vi "mqttTCPIPserver.vi"(0 "mqtt.lvclass":refnum<class "mqtt.lvclass">, 11 "error in (no error)":errorcluster) -> (4 "mqtt.lvclass 2":refnum<class "mqtt.lvclass">, 15 "error out":errorcluster)   [LabVIEW 2018, in "labview-mqtt.lvlib" / "mqtt.lvclass"]
uses:
  mqtt.lvclass
  mqtt.lvclass/mqtt.ctl
  mqttTypedef/mqttRXdataCluster.ctl
  mqttTypedef/mqttFixedHeaderResponse.ctl
  mqttTypedef/mqttQOSlevel.ctl
  mqttTypedef/mqttMessageType.ctl
  mqttTypedef/mqttRXsubscriptionEventData.ctl
  labview-mqtt.lvlib
  mqttCmd/mqttCmdPublish/mqttCmdPublish.lvclass
  mqttCmd/mqttCmdPing/mqttCmdPing.lvclass
panel:
  out "rxCount":i32
  out "rxTelegram":u8[](array[numeric]) format="%02x"
  out "txError":errorcluster
  out "txTelegram":u8[](array[numeric]) format="%02x"
  out "payloadError":errorcluster
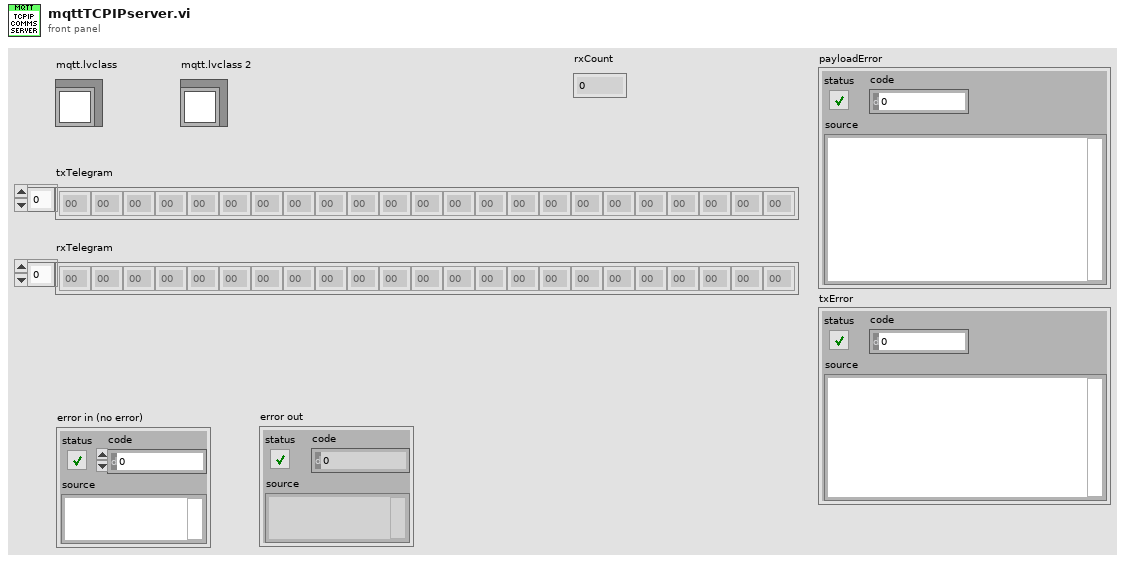
[diagram p1: front panel]
types:
  T1 = typedef "labview-mqtt.lvlib/mqttRXdataCluster.ctl" = cluster{"fixedHdr":T2, "payload":u8[]}
  T2 = typedef "labview-mqtt.lvlib/mqttFixedHeaderResponse.ctl" = cluster{"retain":bool, "qos":T3, "duplicate":bool, "response":T4}
  T3 = typedef "labview-mqtt.lvlib/mqttQOSlevel.ctl" = enum8{"At most once", "At least once", "Exactly once", "Reserved"}
  T4 = typedef "labview-mqtt.lvlib/mqttMessageType.ctl" = enum32{"Reserved", "CONNECT", "CONNACK", "PUBLISH", "PUBACK", "PUBREC", "PUBREL", "PUBCOMP", "SUBSCRIBE", "SUBACK", "UNSUBSCRIBE", "UNSUBACK", "PINGREQ", "PINGRESP", "DISCONNECT", "Reserved2"}
  T5 = typedef "labview-mqtt.lvlib/mqttRXsubscriptionEventData.ctl" = cluster{"topic":string, "value":string, "messageID":u16}
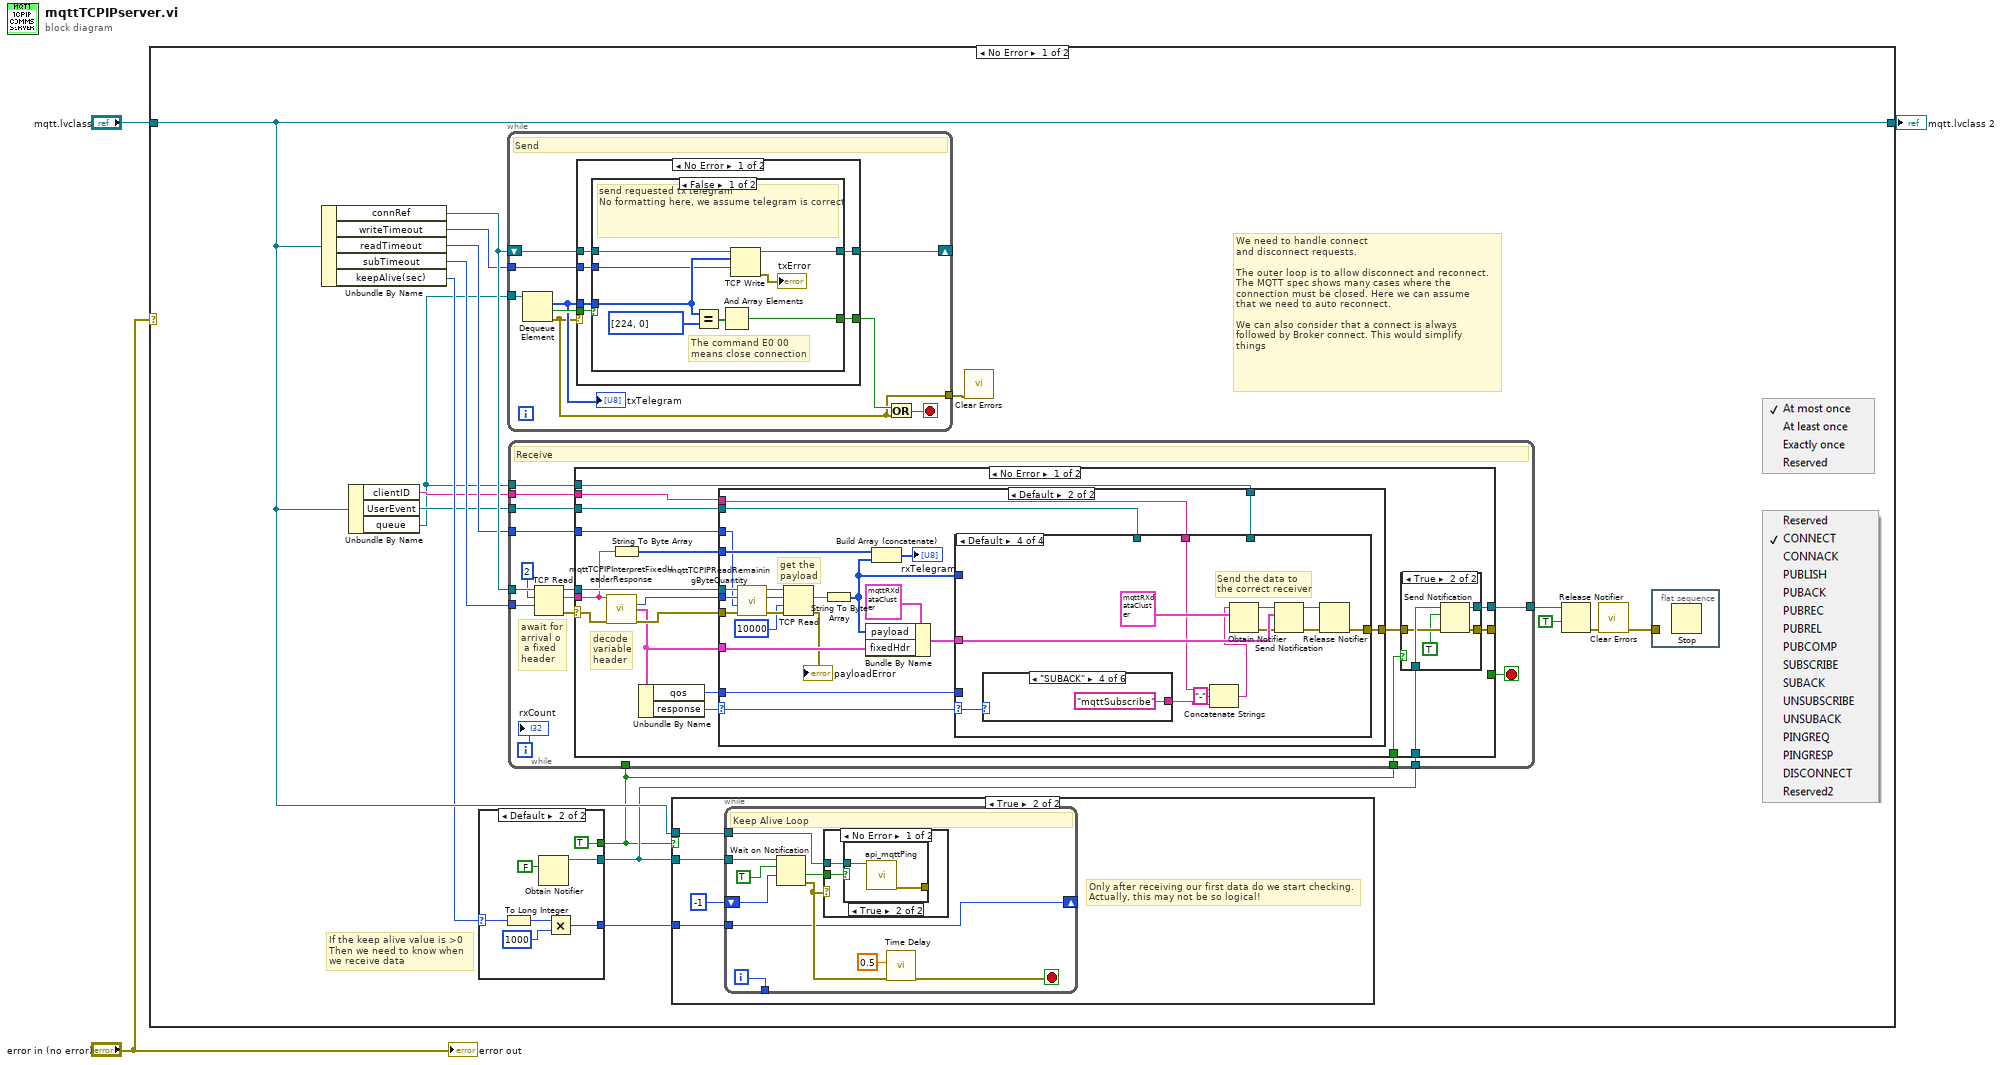
[diagram p0: block diagram]
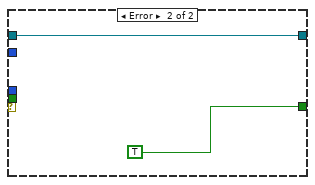
[diagram p7: hidden frame]
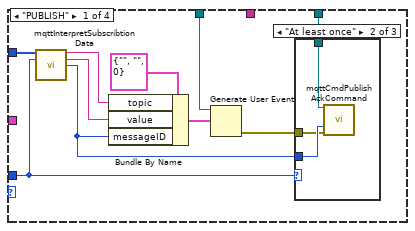
[diagram p10: hidden frame]
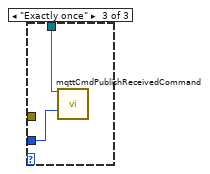
[diagram p12: hidden frame]
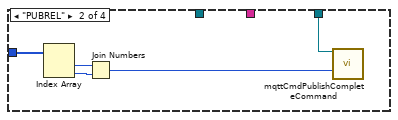
[diagram p13: hidden frame]
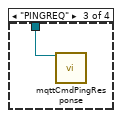
[diagram p14: hidden frame]
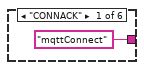
[diagram p15: hidden frame]
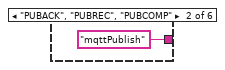
[diagram p16: hidden frame]
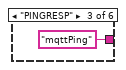
[diagram p17: hidden frame]
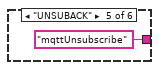
[diagram p18: hidden frame]
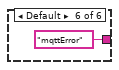
[diagram p19: hidden frame]
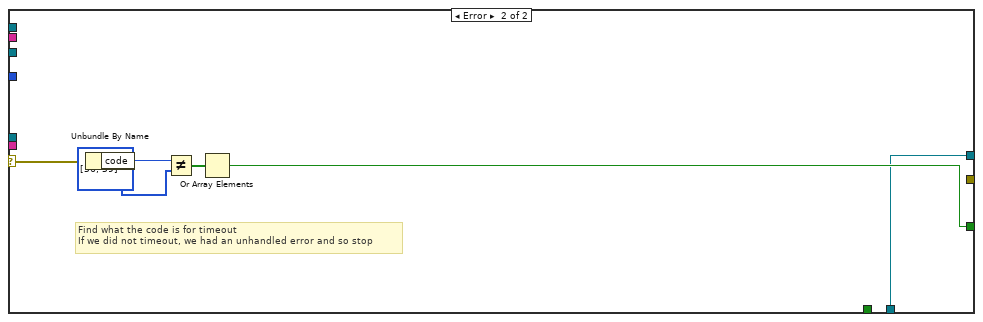
[diagram p20: hidden frame]
diagram:
  n1 = case shown="No Error" "error in (no error)" {
    tunnel: "mqtt.lvclass" -> [w20 w177]
    tunnel: [w20 w177] -> w2
    frame No Error {
      # "If the keep alive value is >0\nThen we need to know when\nwe receive data"
      # "We need to handle connect\nand disconnect requests.\n\nThe outer loop is to allow disconnect and reconnect.\nThe MQTT spec shows many cases where the\nconnection must be closed. Here we can assume\nthat we need to auto reconnect.\n\nWe can also consider that a connect is always\nfollowed by Broker connect. This would simplify\nthings"
      n2 = Unbundle By Name(w20) -> ("connRef"=w19:refnum<k5>, "writeTimeout"=w17:i32, "readTimeout"=w16:i32, "subTimeout"=w15:i32, "keepAlive(sec)"=w9:u16)
      n3 = Unbundle By Name(w20) -> ("clientID"=w6:string, "UserEvent"=w7:refnum<user-event>, "queue"=w5:refnum<queue>)
      n4 = case shown="Default" w9 {
        selector: w9 -> [_ w40]
        tunnel: [_ w45] -> w14
        tunnel: [_ w41] -> w10
        tunnel: [_ TRUE] -> w8
        frame ..0 {
        }
        frame Default {
          n5 = To Long Integer(number=w40) -> (32bit integer=w43:i32)
          n6 = Obtain Notifier(notification data type=FALSE) -> (notifier out=w45:refnum<notifier>)  [unwired: 3 in, 2 out]
          n7 = Multiply(x=w43, y=1000) -> (x*y=w41:i32)
        }
      }
      n8 = while {
        tunnel: w5 -> [w54]
        shift-right: [w51] -> _
        shift-left: w19 -> [w52]
        tunnel: [w47] -> w18
        tunnel: w17 -> [w46]
        stop <- w50 stop-if-true
        # "Send"
        n9 = Dequeue Element(queue=w54) -> (element=w48:u8[], timed out?=w53:bool, error out=w47:errorcluster)  [unwired: 2 in, 1 out]
        "txTelegram" <- w48
        n10 = case shown="No Error" w47 {
          tunnel: w53 -> [w60 _]
          tunnel: w48 -> [w59 _]
          tunnel: w52 -> [w58 w71]
          tunnel: [w57 w71] -> w51
          tunnel: [w56 TRUE] -> w49
          tunnel: w46 -> [w55 _]
          frame No Error {
            n11 = case shown="False" w60 {
              tunnel: w59 -> [w66 _]
              tunnel: w58 -> [w68 w69]
              tunnel: [w67 w69] -> w57
              tunnel: [w63 _] -> w56
              tunnel: w55 -> [w61 _]
              frame False {
                # "The command E0 00\nmeans close connection"
                # "send requested tx telegram\nNo formatting here, we assume telegram is correct"
                n12 = Equal?(x=w66, y=u8[] [224, 0] ("txTelegram 2")) -> (x = y?=w64:bool[])
                n13 = And Array Elements(Boolean array=w64) -> (logical AND=w63:bool)
                n14 = TCP Write(connection ID=w68, data in=w66, 9:w61) -> (connection ID out=w67:refnum<k5>, error out=→"txError":errorcluster)  [unwired: 1 in, 1 out]
              }
              frame True {
                # "Queue Timed Out - do nothing.\nWe can later use this for the Keep Alive ping"
              }
            }
          }
          frame Error {
          }
        }
        n15 = Or(x=w49, y=w47) -> (x .or. y?=w50:bool)
      }
      n16 = while {
        tunnel: w19 -> [w86]
        tunnel: w16 -> [w79]
        tunnel: w15 -> [w78]
        tunnel: w14 -> [w77]
        tunnel: [w76] -> w13
        tunnel: w8 -> [w75]
        tunnel: w8 -> [_]
        tunnel: w7 -> [w74]
        tunnel: w5 -> [w73]
        tunnel: w6 -> [w72]
        i -> [w80]
        stop <- w81 stop-if-true
        # "await for\narrival o\n a fixed\nheader"
        # "Receive"
        n17 = TCP Read(connection ID=w86, bytes to read=2, 9:w78) -> (connection ID out=w85:refnum<k5>, data out=w82:string, error out=w84:errorcluster)  [unwired: 2 in]
        n18 = case shown="No Error" w84 {
          selector: w84 -> [w102 w176]
          tunnel: w85 -> [w103 _]
          tunnel: w82 -> [w98 _]
          tunnel: [_ w172] -> w81
          tunnel: w79 -> [w95 _]
          tunnel: w77 -> [w94 w171]
          tunnel: [w92 w171] -> w76
          tunnel: [w91 _] -> _
          tunnel: w75 -> [w90 _]
          tunnel: w74 -> [w89 _]
          tunnel: w73 -> [w88 _]
          tunnel: w72 -> [w87 _]
          frame No Error {
            # "decode\nvariable\nheader"
            n19 = call "mqttTCPIPInterpretFixedHeaderResponse.vi"("data in"=w98, "error in (no error)"=w102) -> ("remainingLengthByte1"=w104:u8, "output cluster"=w100:T2, "error out"=w101:errorcluster)  [unwired: 11 in]
            n20 = String To Byte Array(string=w98) -> (unsigned byte array=w97:u8[])
            n21 = Unbundle By Name(w100) -> ("qos"=w96:T3, "response"=w99:T4)
            n22 = case shown="Default" w99 {
              selector: w99 -> [_ w121]
              tunnel: w104 -> [_ w131]
              tunnel: w103 -> [_ w130]
              tunnel: w101 -> [_ w123]
              tunnel: w100 -> [_ w122]
              tunnel: w97 -> [_ w118]
              tunnel: w96 -> [_ w117]
              tunnel: w95 -> [_ w114]
              tunnel: [_ w113] -> w93
              tunnel: w89 -> [_ w112]
              tunnel: w88 -> [_ w111]
              tunnel: w87 -> [_ w110]
              frame "CONNECT", "SUBSCRIBE" {
                # "The client should not receive these commands.\nI had some problems with these commands being received\nand it appears this was a broker issue. However, to ignore\nmessages that we should not receive is no bad thing."
              }
              frame Default {
                # "get the\npayload"
                n23 = call "mqttTCPIPReadRemainingByteQuantity.vi"("error in (no error)"=w123, "readTimeout ms (2000)"=w114, "remainingLengthByte1"=w131, "connRef in"=w130) -> ("error out"=w128:errorcluster, "remainingLength"=w127:i32, "connRef out"=w129:refnum<k5>)  [unwired: 5 in]
                n24 = TCP Read(connection ID=w129, bytes to read=w127, error in (no error)=w128, 9:10000 ("timeout ms (25000)")) -> (data out=w125:string, error out=→"payloadError":errorcluster)  [unwired: 1 in, 1 out]
                n25 = String To Byte Array(string=w125) -> (unsigned byte array=w115:u8[])
                n26 = Bundle By Name(cluster=T1 {"fixedHdr"={"retain"=FALSE, "qos"=enum."At most once", "duplicate"=FALSE, "response"=enum."Reserved"}, "payload"=[]} ("output cluster"), "payload"=w115, "fixedHdr"=w122) -> (w119:T1)
                n27 = Build Array (concatenate)(w118, w115) -> (→"rxTelegram":u8[])
                n28 = case shown="Default" w121 {
                  selector: w121 -> [_ _ _ w164]
                  tunnel: w119 -> [_ _ _ w163]
                  tunnel: w117 -> [w137 _ _ _]
                  tunnel: w115 -> [w140 w151 _ _]
                  tunnel: [_ _ _ w153] -> w113
                  tunnel: w112 -> [w134 _ _ _]
                  tunnel: w111 -> [w132 w147 w152 _]
                  tunnel: w110 -> [_ _ _ w159]
                  frame "PUBLISH" {
                    n29 = call "mqttInterpretSubscribtionData.vi"("rxTelegram in"=w140, "qos"=w137) -> ("topic"=w139:string, "value"=w138:string, "messageID"=w136:u16)  [unwired: 10 in, 1 out]
                    n30 = Bundle By Name(cluster=T5 {"topic"="", "value"="", "messageID"=0} ("data"), "topic"=w139, "value"=w138, "messageID"=w136) -> (w133:T5)
                    n31 = Generate User Event(user event=w134, event data cluster=w133) -> (error out=w135:errorcluster)  [unwired: 2 in, 1 out]
                    n32 = case shown="\"At least once\"" w137 {
                      tunnel: w136 -> [_ w144 w146]
                      tunnel: w135 -> [_ w143 _]
                      tunnel: w132 -> [_ w142 w145]
                      frame Default {
                      }
                      frame "At least once" {
                        n33 = call "mqttCmdPublishAckCommand.vi"("queue"=w142, "messageID"=w144, "error in (no error)"=w143) -> ()  [unwired: 12 in, 1 out]
                      }
                      frame "Exactly once" {
                        n34 = call "mqttCmdPublishReceivedCommand.vi"("queue"=w145, "messageID"=w146) -> ()  [unwired: 13 in, 1 out]
                      }
                    }
                  }
                  frame "PUBREL" {
                    n35 = Index Array(array=w151) -> (element #1=w150:u8, element #2=w149:u8)  [unwired: 2 in]
                    n36 = Join Numbers(hi=w150, lo=w149) -> ((hi.lo)=w148:u16)
                    n37 = call "mqttCmdPublishCompleteCommand.vi"("queue"=w147, "messageID"=w148) -> ()  [unwired: 13 in, 1 out]
                  }
                  frame "PINGREQ" {
                    n38 = call "mqttCmdPingResponse.vi"("queue"=w152) -> ()  [unwired: 14 in, 1 out]
                  }
                  frame Default {
                    # "Send the data to\nthe correct receiver"
                    n39 = case shown="\"SUBACK\"" w164 {
                      tunnel: ["mqttConnect" ("name (unnamed)") "mqttPublish" ("name (unnamed)") "mqttPing" ("name (unnamed)") "mqttSubscribe" ("name (unnamed)") "mqttUnsubscribe" ("name (unnamed)") "mqttError" ("name (unnamed)")] -> w157
                      frame "CONNACK" {
                      }
                      frame "PUBACK", "PUBREC", "PUBCOMP" {
                      }
                      frame "PINGRESP" {
                      }
                      frame "SUBACK" {
                      }
                      frame "UNSUBACK" {
                      }
                      frame Default {
                      }
                    }
                    n40 = Concatenate Strings(w159, "-" ("string"), w157) -> (w156:string)
                    n41 = Obtain Notifier(name (unnamed)=w156, notification data type=T1 {"fixedHdr"={"retain"=FALSE, "qos"=enum."At most once", "duplicate"=FALSE, "response"=enum."Reserved"}, "payload"=[]} ("output cluster")) -> (notifier out=w162:refnum<notifier>, error out=w160:errorcluster)  [unwired: 2 in, 1 out]
                    n42 = Send Notification(notification=w163, notifier=w162, error in (no error)=w160) -> (notifier out=w154:refnum<notifier>, error out=w155:errorcluster)
                    n43 = Release Notifier(notifier=w154, error in (no error)=w155) -> (error out=w153:errorcluster)  [unwired: 1 in, 2 out]
                  }
                }
              }
            }
            n44 = case shown="True" w90 {
              tunnel: w94 -> [_ w109]
              tunnel: w93 -> [_ w108]
              tunnel: [_ w106] -> w92
              tunnel: [_ w105] -> w91
              frame False {
              }
              frame True {
                n45 = Send Notification(notification=TRUE, notifier=w109, error in (no error)=w108) -> (notifier out=w106:refnum<notifier>, error out=w105:errorcluster)
              }
            }
          }
          frame Error {
            # "Find what the code is for timeout\nIf we did not timeout, we had an unhandled error and so stop"
            n46 = Unbundle By Name(w176) -> ("code"=w175:i32)
            n47 = Not Equal?(x=w175, y=i32[] [56, 59]) -> (x != y?=w173:bool[])
            n48 = Or Array Elements(Boolean array=w173) -> (logical OR=w172:bool)
          }
        }
        "rxCount" <- w80
      }
      n49 = case shown="True" w8 {
        tunnel: w14 -> [_ w24]
        tunnel: w10 -> [_ w23]
        tunnel: w20 -> [_ w21]
        frame False {
        }
        frame True {
          # "Only after receiving our first data do we start checking.\nActually, this may not be so logical!"
          n50 = while {
            tunnel: w24 -> [w34]
            tunnel: [w29] -> _
            shift-right: [w26] -> _
            shift-left: -1 -> [w33]
            tunnel: w23 -> [w26]
            tunnel: w21 -> [w25]
            i -> [w29]
            stop <- w30 stop-if-true
            # "Keep Alive Loop"
            n51 = Wait on Notification(notifier=w34, ignore previous (F)=TRUE, timeout in ms (-1)=w33) -> (timed out?=w32:bool, error out=w27:errorcluster)  [unwired: 1 in, 2 out]
            n52 = case shown="No Error" w27 {
              tunnel: w32 -> [w36 _]
              tunnel: w25 -> [w35 _]
              frame No Error {
                n53 = case shown="True" w36 {
                  tunnel: [_ w38] -> _
                  tunnel: w35 -> [_ w37]
                  frame False {
                  }
                  frame True {
                    n54 = call "api_mqttPing.vi"("mqtt.lvclass in"=w37) -> ("error out"=w38:errorcluster)  [unwired: 12 in, 2 out]
                  }
                }
              }
              frame Error {
              }
            }
            n55 = call "Time Delay"("error in (no error)"=w27, "Delay Time (s)"=0.5) -> ("error out"=w30:errorcluster)  [unwired: 9 in]
          }
        }
      }
      n56 = call <vilib>:"Clear Errors.vi"("error in (no error)"=w18) -> ()  [unwired: 5 in, 2 out]
      n57 = Release Notifier(notifier=w13, force destroy? (F)=TRUE) -> (error out=w11:errorcluster)  [unwired: 1 in, 2 out]
      n58 = call <vilib>:"Clear Errors.vi"("error in (no error)"=w11) -> ("error out"=w4:errorcluster)  [unwired: 5 in, 1 out]
      n59 = flat-sequence {
        tunnel: w4 -> [_]
        frame #0 {
          n60 = Stop() -> ()  [unwired: 1 in]
        }
      }
    }
    frame Error {
    }
  }
  "mqtt.lvclass 2" <- w2
  "error out" <- "error in (no error)"
